vi "RT Main_Read Scalar.vi"() -> ()   [LabVIEW 2018]
uses:
  <vilib>/Platform/TimedLoop/XDataNode/timing_clust.ctl
  <vilib>/Platform/TimedLoop/XDataNode/nitl_modes.ctl
  <vilib>/Platform/TimedLoop/XDataNode/wakeup.ctl
  FPGA Bitfile Register Operations/Scalar IO Operations/TypeDefs/FXP Configuration.ctl
  <vilib>/fxp/LVFixedPointRepBitsTypeDef.ctl
  <vilib>/fxp/LVFixedPointRepRangeTypeDef.ctl
  FPGA Bitfile Register Operations/Scalar IO Operations/Read Methods/Read Data Register/Instances/Read FXP.vi
  FPGA Bitfile Register Operations/Scalar IO Operations/SubVIs/FXP Raw to DBL.vi
  FPGA Bitfile Register Operations/Scalar IO Operations/Read Methods/Read Data Register/Instances/Read U16.vi
  FPGA Bitfile Register Operations/Scalar IO Operations/Read Methods/Read Data Register/Instances/Read U32.vi
  FPGA Bitfile Register Operations/Scalar IO Operations/Read Methods/Read Data Register/Instances/Read U64.vi
  FPGA Bitfile Register Operations/Scalar IO Operations/Read Methods/Read Data Register/Instances/Read U8.vi
  FPGA Bitfile Register Operations/Scalar IO Operations/Utilities/Find Register Offset.vi
  FPGA Bitfile Register Operations/Scalar IO Operations/SubVIs/Check Register Data Store.vi
  FPGA Bitfile Register Operations/Scalar IO Operations/Error Handling/Error 6001.vi
  FPGA Bitfile Register Operations/Scalar IO Operations/Error Handling/Error 6000.vi
  FPGA Bitfile Register Operations/Scalar IO Operations/Error Handling/Error 6002.vi
  FPGA Bitfile Register Operations/Scalar IO Operations/Error Handling/Error 6003.vi
  <vilib>/FPGAPlugInAG/Dynamic/niLvFpga_Close_Dynamic.vi
  <vilib>/platform/TimedLoop/XDataNode/XDataNode.xnode
  <vilib>/rvi/interface/nirviCloseFPGA/nirviCloseFPGA.xnode
  FPGA Bitfile Register Operations/Scalar IO Operations/FPGA Register IO.lvlib
  <vilib>/Platform/TimedLoop/XDataNode/XDNodeRunTimeDep.lvlib
panel:
  out "DBL Value Out":dbl format="%#.6g"
  out "Average seconds per read":dbl format="%#_6e"
  out "error out":errorcluster
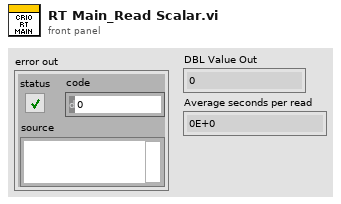
[diagram p1: front panel]
types:
  T1 = typedef "XDNodeRunTimeDep.lvlib/timing_clust.ctl" = cluster{"Expected End [f-1]":u64, "Actual End [f-1]":u64, "Finished Late? [f-1]":bool, "Expected End [i-1]":u64, "Actual End [i-1]":u64, "Finished Late? [i-1]":bool, "Expected Start [i]":u64, "Actual Start [i]":u64, "Expected Start [f]":u64, "Actual Start [f]":u64, "Source Name":string, "Structure Name":string, "Period":i64, "Deadline":i64, "Offset":i64, "Start":i64, "Priority":i32, "Timeout":i32, "Mode":T2, "Wakeup Reason":T3, "Error":errorcluster, "Source Type":string, "Secondary Source Type":string, "Global End Time":u64, "Global Start Time":u64, "Frame Duration":u64, "Iteration Duration":u64, "Assigned CPU":i32, "I/O Scan Engine Mode":u32}
  T2 = typedef "XDNodeRunTimeDep.lvlib/nitl_modes.ctl" = enum32{"No Change", "Process missed periods, maintain original phase", "Discard missed periods, maintain original phase", "Process missed periods, ignore original phase", "Discard missed periods, ignore original phase"}
  T3 = typedef "XDNodeRunTimeDep.lvlib/wakeup.ctl" = enum32{"Normal", "Aborted", "Asynchronous wakeup", "Timing source error", "Timed loop error", "Timeout"}
  T4 = typedef "FPGA Register IO.lvlib/FXP Configuration.ctl" = cluster{"FXP Representation":T5, "FXP Range":T6}
  T5 = typedef "LVFixedPointRepBitsTypeDef.ctl" = cluster{"Signed":bool, "Word Length":u32, "Integer Word Length":i32}
  T6 = typedef "LVFixedPointRepRangeTypeDef.ctl" = cluster{"Range Min":dbl, "Range Max":dbl, "Delta":dbl}
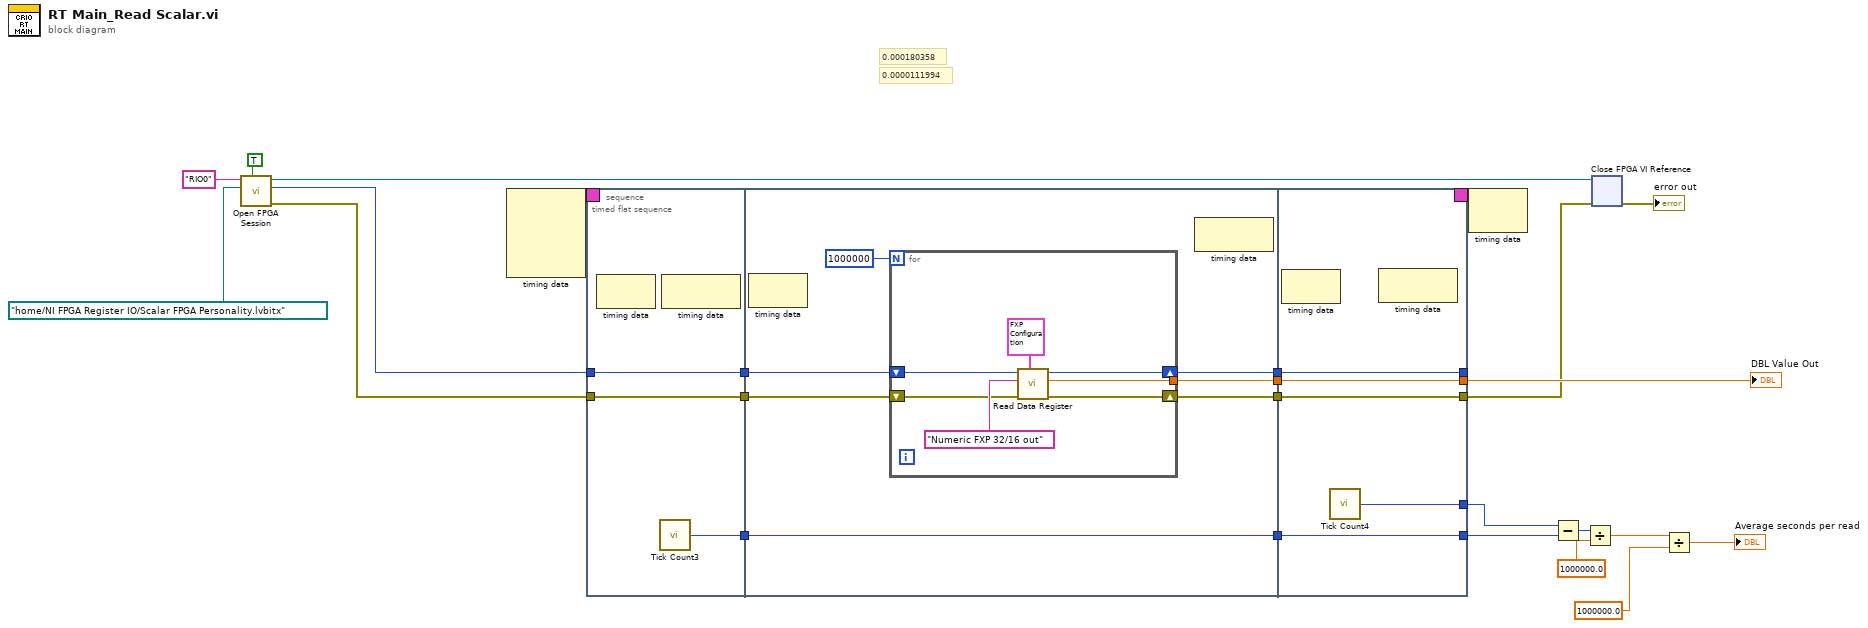
[diagram p0: block diagram]
diagram:
  # "0.0000111994"
  # "0.000180358"
  n1 = call "Open FPGA Session.vi"("run when loaded (T)"=TRUE ("Run When Loaded (T)"), "bitfile path"=path "/home/NI FPGA Register IO/Scalar FPGA Personality.lvbitx" ("Bitfile path"), "device address"="RIO0" ("Device address")) -> ("error out"=w9:errorcluster, "session out"=w10:u32, "bitfile reference out"=w12:refnum<k20>)  [unwired: 6 in]
  n2 = node-c288() -> (w18:T1)  [unwired: 4 in]
  n3 = timed-sequence {
    timing: w18 -> [_]
    timing-out: [_] -> w17
    tunnel: w10 -> [w32]
    tunnel: w9 -> [w31]
    tunnel: [w26] -> w8
    tunnel: [w25] -> w7
    tunnel: [w24] -> _
    tunnel: [w21] -> w1
    tunnel: [w19] -> w2
    n4 = timed-flat-sequence {
      tunnel: w31 -> [w34]
      tunnel: w32 -> [w35]
      tunnel: [w35] -> w30
      tunnel: [w34] -> w29
      tunnel: [w33] -> w28
      tunnel: w30 -> [w44]
      tunnel: w29 -> [w43]
      tunnel: w28 -> [w41]
      tunnel: [w41] -> w27
      tunnel: [w40] -> w23
      tunnel: [w39] -> w22
      tunnel: [w38] -> w20
      tunnel: w27 -> [w57]
      tunnel: [w58] -> w26
      tunnel: [w57] -> w25
      tunnel: [w56] -> w24
      tunnel: w23 -> [w56]
      tunnel: w22 -> [w55]
      tunnel: [w55] -> w21
      tunnel: w20 -> [w54]
      tunnel: [w54] -> w19
      frame #0 {
        n5 = node-c288() -> ()  [unwired: 1 in, 1 out]
        n6 = call "Tick Count3"() -> ("Tick Count(uSec)"=w33:u32)
        n7 = node-c288() -> ()  [unwired: 1 in, 1 out]
      }
      frame #1 {
        n8 = node-c288() -> ()  [unwired: 1 in, 1 out]
        n9 = for {
          N: 1000000 -> [_]
          shift-right: [w47] -> w39
          shift-left: w43 -> [w50]
          shift-right: [w48] -> w40
          shift-left: w44 -> [w49]
          tunnel: [w45] -> w38
          n10 = call-poly "Read Data Register.vi"("FXP Configuration"=T4 {"FXP Representation"={"Signed"=TRUE, "Word Length"=32, "Integer Word Length"=16}, "FXP Range"={"Range Min"=0.0, "Range Max"=0.0, "Delta"=1.52588e-05}}, "error in"=w50, "register name"="Numeric FXP 32/16 out", "session in"=w49) -> ("error out"=w47:errorcluster, "DBL Value"=w45:dbl, "session out"=w48:u32)  [unwired: 5 in]
        }
        n11 = node-c288() -> ()  [unwired: 1 in, 1 out]
      }
      frame #2 {
        n12 = node-c288() -> ()  [unwired: 1 in, 1 out]
        n13 = call "Tick Count4"() -> ("Tick Count(uSec)"=w58:u32)
        n14 = node-c288() -> ()  [unwired: 1 in, 1 out]
      }
    }
  }
  "DBL Value Out" <- w2
  n15 = node-c288(w17) -> ()  [unwired: 1 out]
  n16 = Subtract(x=w8, y=w7) -> (x-y=w6:u32)
  n17 = Divide(x=w6, y=1000000.0) -> (x/y=w5:dbl)
  n18 = xnode "Close FPGA VI Reference"("FPGA VI Reference In"=w12, "error in"=w1) -> ("error out"=→"error out":errorcluster)
  n19 = Divide(x=w5, y=1000000.0) -> (x/y=→"Average seconds per read":dbl)
